vi "系统设置.vi"() -> ()   [LabVIEW 2016]
uses:
  PLC/control/switch.ctl
  <vilib>/Utility/miscctls.llb/LVPointTypeDef.ctl
  API/Alarm interface/interface.vi
  API/DGUS/SourceCode/DGUS/Interface/task.vi
  <vilib>/ptbypt/NI_PtbyPt.lvlib
  <vilib>/Utility/config.llb/NI_LVConfig.lvlib
  PLC/PLC.lvlib
  API/Alarm interface/Alarm interface.lvlib
  API/OpSignIn/opSignIn.lvlib
  API/DGUS/SourceCode/DGUS.lvlib
panel:
  in  "更新数据库密码":bool
  in  "性能测试模式":bool
  in  "运维打卡配置":bool
  in  "平行样测试":T1
  in  "采水模式":enum16{"单采水点", "交替采水"}(ring)
  in  "停止":T1
  in  "集成干预测试":T1
  out "最近一次启动时间":string
  in  "单次水样测试":T1
  in  "站点信息设置":bool
  in  "自动运行启动参数":T2
  in  "定时重启配置":bool
  in  "模块启用配置":bool
  in  "报警设置":bool
  in  "首页显示设置":bool
  in  "跨度核查":T1
  in  "零点核查":T1
  out "选项卡控件":enum32{"自由设定", "国标协议", "流量设定"}(tab)
  in  "24H周期设置":T3
  in  "采配水运行间隔":i16=4 min=0 max=24
  in  "多参数运行间隔":i16=4 min=0 max=24
  in  "湿化学运行间隔":i16=4 min=0 max=24
  in  "流量阈值":dbl=4.0 min=1.0 max=24.0
  in  "时间阈值":u16=4 min=1 max=24
  in  "周期设置":enum16{"自由设定", "国标协议", "流量设定"}(ring)
  in  "质控启动日期":string(combo)="关闭"
  in  "跨度核查时间":u16(ring)=6 items=["00H", "01H", "02H", "03H", "04H", "05H", "06H", "07H", "08H", "09H", "10H", "11H", "12H", "13H", "14H", "15H", "16H", "17H", "18H", "19H", "20H", "21H", "22H", "23H", "关闭"]
  in  "空白核查时间":u16(ring)=2 items=["00H", "01H", "02H", "03H", "04H", "05H", "06H", "07H", "08H", "09H", "10H", "11H", "12H", "13H", "14H", "15H", "16H", "17H", "18H", "19H", "20H", "21H", "22H", "23H", "关闭"]
  in  "副屏显示设置":bool
  in  "开机启动":bool caption="氨氮禁用"
  in  "运行模式":enum16{"维护模式", "常规模式", "应急模式", "质控模式"}(ring)
  # "注：周期设置分为自由设定和国标协议两种。\n1：选择自由设定情况下：运行间隔将不可选用并变灰色，周期设置可自由手动勾选\n2：选择国标协议情况下：周期时间将由运行间隔选择的时间决定，下方周期设置被禁用并无法手动勾选。\n3：选择流量设定情况下：瞬时流量连续超过流量阈值到达时间阈值设定值，仪器将自动开启测量。"
  # "质控频次："
  # "零点核查时间："
  # "跨度核查时间："
  # "启动周期设置"
  # "采水模式：\n单采水点：依据采水泵模式启动采水泵\n交替采水：采水泵根据周期设置交替启动"
  # "m3/S"
  # "秒"
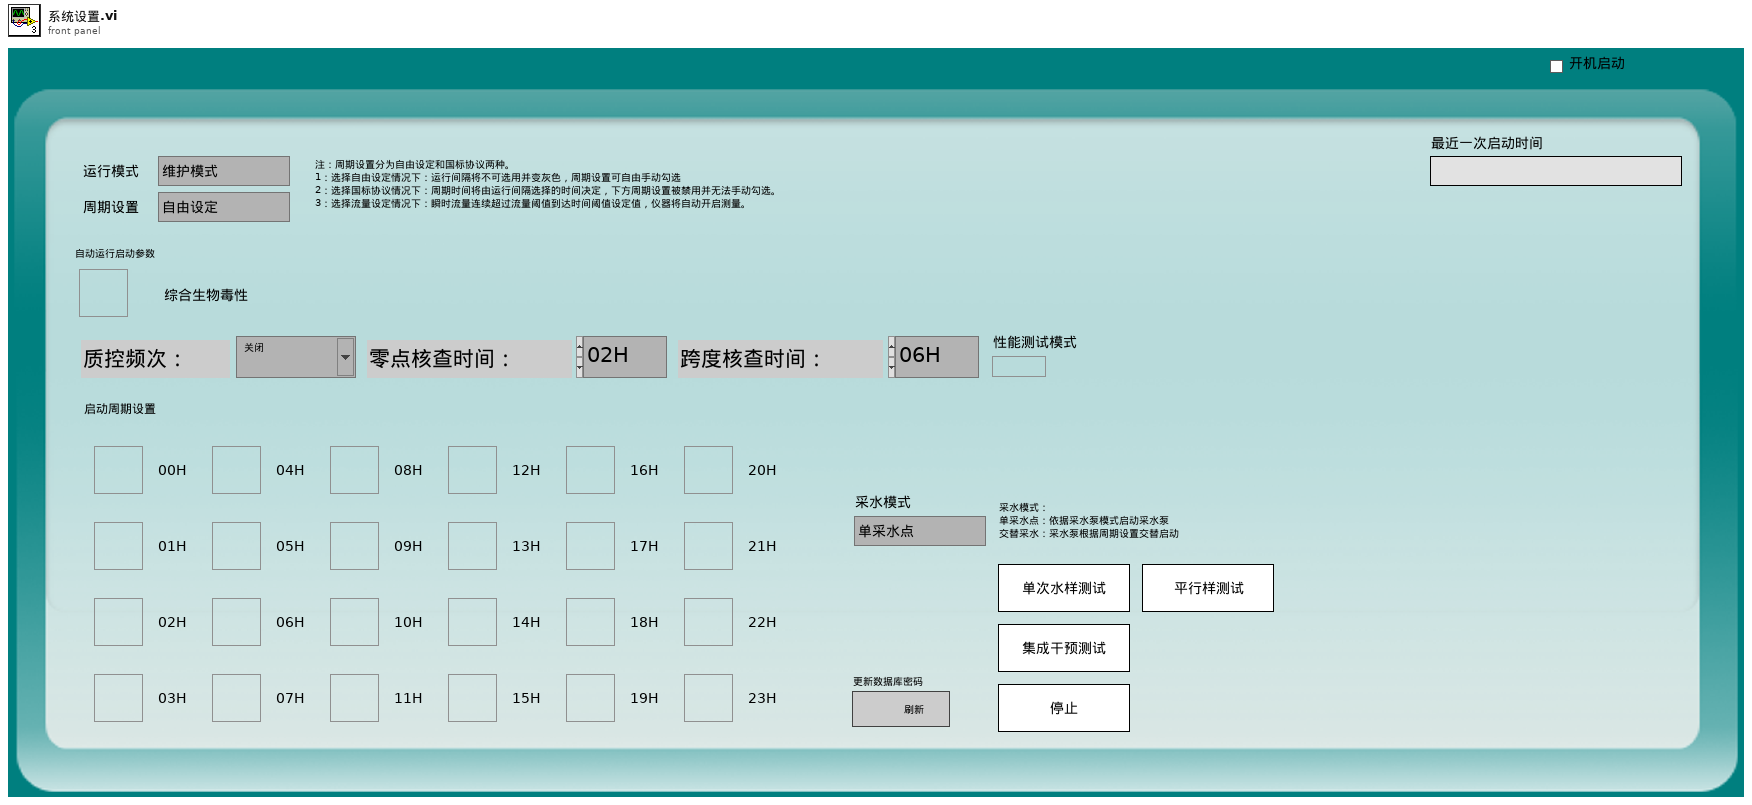
[diagram p1: front panel]
types:
  T1 = typedef "PLC.lvlib/switch.ctl" = bool
  T2 = typedef "启动参数.ctl" = cluster{"氨氮":bool, "总磷":bool, "总氮":bool, "多参数":bool, "CODmn":bool, "CODCr":bool, "氟化物":bool, "超标留样":bool, "重金属":bool, "挥发酚":bool, "综合生物毒性":bool}
  T3 = typedef "24周期设置.ctl" = cluster{"00H":bool, "01H":bool, "02H":bool, "03H":bool, "04H":bool, "05H":bool, "06H":bool, "07H":bool, "08H":bool, "09H":bool, "10H":bool, "11H":bool, "12H":bool, "13H":bool, "14H":bool, "15H":bool, "16H":bool, "17H":bool, "18H":bool, "19H":bool, "20H":bool, "21H":bool, "22H":bool, "23H":bool}
  T4 = cluster{"控制命令":enum16{"启动测量", "标样核查", "零点核查", "跨度核查", "空白测试", "平行样测试", "加标回收", "空白校准", "标样校准", "初始化（清洗）", "停止测试", "仪器重启", "校时", "模式设置", "测量间隔设置"}, "自动运行启动参数":T2}
  T5 = typedef "参数.ctl" = cluster{"测试模式":enum16{"水样测试", "平行样测试", "集成干预测试", "加标回收"}, "参数启用":T2}
  T6 = typedef "LVPointTypeDef.ctl" = cluster{"Horizontal":i16, "Vertical":i16}
  T7 = enum8{"Enabled", "Disabled", "Disabled and Grayed Out"}
  T8 = cluster{"频次":enum16{"关闭", "每天", "星期一", "星期二", "星期三", "星期四", "星期五", "星期六", "星期日"}, "时":u16, "分":u16}
  T9 = typedef "LVDateTimeRec.ctl" = cluster{"秒数的小数部分":dbl, "秒":i32, "分":i32, "时":i32, "日":i32, "月":i32, "年":i32, "天数（周）":i32, "天数（年）":i32, "DST":i32}
  T10 = enum16{"关闭", "每天", "星期一", "星期二", "星期三", "星期四", "星期五", "星期六", "星期日"}
  T11 = enum32{"Bad", "Idle", "Run top level", "Running"}
  T12 = enum32{"Invalid", "Standard", "Closed", "Hidden", "Minimized", "Maximized"}
  T13 = typedef "LVAllMonitorsDisplayTypeDef.ctl" = cluster{"Bounds":cluster{"Left":i16, "Top":i16, "Right":i16, "Bottom":i16}, "Depth":i16}[]
  T14 = cluster{"24H周期设置[0]":bool, "24H周期设置[1]":bool, "24H周期设置[2]":bool, "24H周期设置[3]":bool, "24H周期设置[4]":bool, "24H周期设置[5]":bool, "24H周期设置[6]":bool, "24H周期设置[7]":bool, "24H周期设置[8]":bool, "24H周期设置[9]":bool, "24H周期设置[10]":bool, "24H周期设置[11]":bool, "24H周期设置[12]":bool, "24H周期设置[13]":bool, "24H周期设置[14]":bool, "24H周期设置[15]":bool, "24H周期设置[16]":bool, "24H周期设置[17]":bool, "24H周期设置[18]":bool, "24H周期设置[19]":bool, "24H周期设置[20]":bool, "24H周期设置[21]":bool, "24H周期设置[22]":bool, "24H周期设置[23]":bool}
  T15 = typedef "操作日志字段定义.ctl" = cluster{"时间":timestamp, "参数":string, "日志信息":string, "流程参数":string}
  T16 = enum16{"启动测量", "标样核查", "零点核查", "跨度核查", "空白测试", "平行样测试", "加标回收", "空白校准", "标样校准", "初始化（清洗）", "停止测试", "仪器重启", "校时", "模式设置", "测量间隔设置"}
  T17 = cluster{"测试模式":enum16{"水样测试", "平行样测试", "集成干预测试", "加标回收"}, "启动参数输出":T2}
  T18 = typedef "NI_LVConfig.lvlib/Config Data RefNum.ctl" = refnum<k1>
  T19 = cluster{"元素":enum16{"启动测量", "标样核查", "零点核查", "跨度核查", "空白测试", "平行样测试", "加标回收", "空白校准", "标样校准", "初始化（清洗）", "停止测试", "仪器重启", "校时", "模式设置", "测量间隔设置"}, "启动参数输出":T2}
  T20 = cluster{"元素":enum16{"启动测量", "标样核查", "零点核查", "跨度核查", "空白测试", "平行样测试", "加标回收", "空白校准", "标样校准", "初始化（清洗）", "停止测试", "仪器重启", "校时", "模式设置", "测量间隔设置"}, "自动运行启动参数":T2}
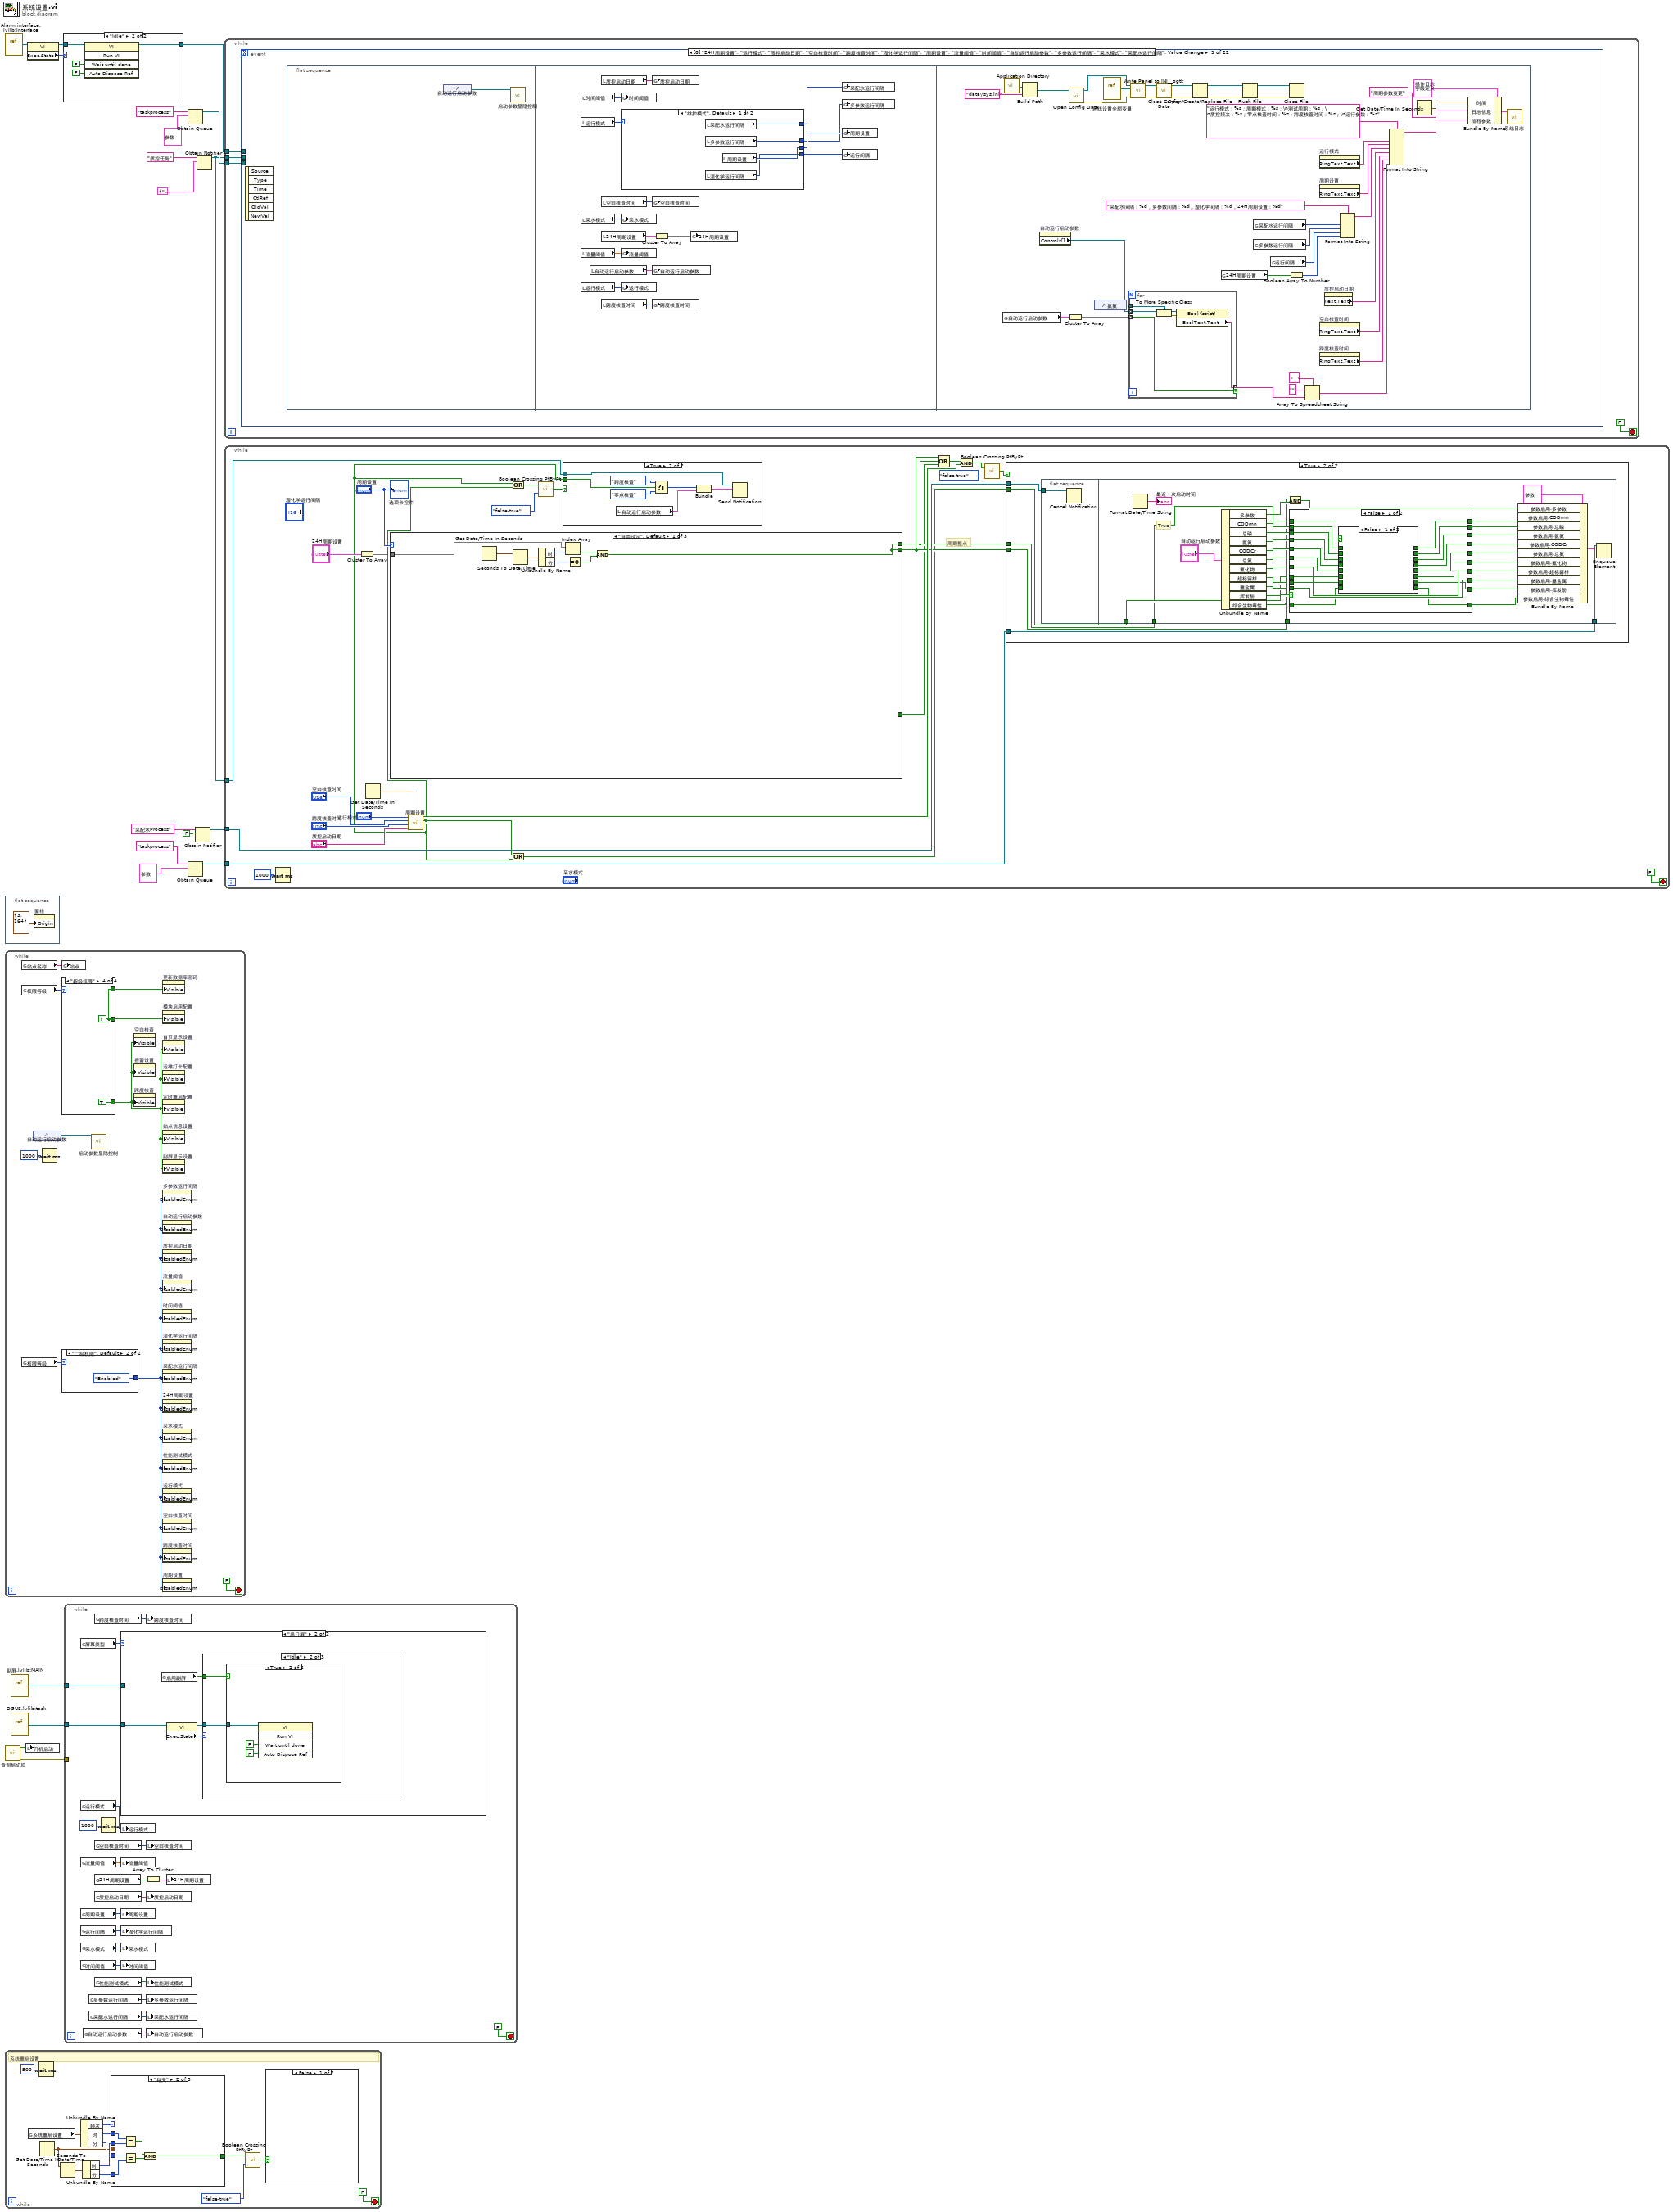
[diagram p0: block diagram]
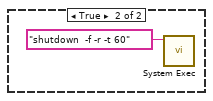
[diagram p2: hidden frame]
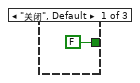
[diagram p3: hidden frame]
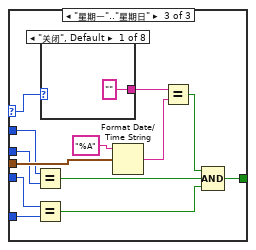
[diagram p4: hidden frame]
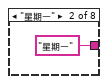
[diagram p5: hidden frame]
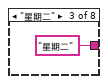
[diagram p6: hidden frame]
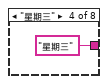
[diagram p7: hidden frame]
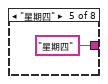
[diagram p8: hidden frame]
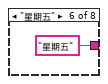
[diagram p9: hidden frame]
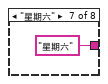
[diagram p10: hidden frame]
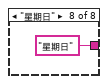
[diagram p11: hidden frame]
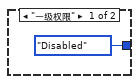
[diagram p13: hidden frame]
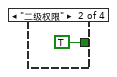
[diagram p15: hidden frame]
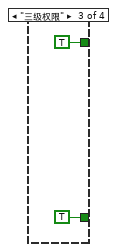
[diagram p16: hidden frame]
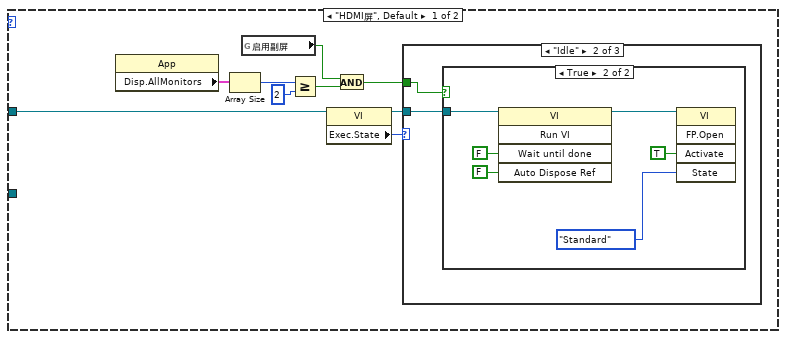
[diagram p17: hidden frame]
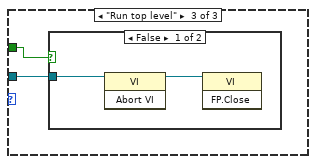
[diagram p20: hidden frame]
diagram:
  n1 = vi-ref "Alarm interface.lvlib:interface.vi"() -> (w15:refnum<vi>)
  n2 = flat-sequence {
    frame #0 {
      n3 = property on="窗格" class="Pane"("Origin"=T6 {"Horizontal"=3, "Vertical"=164} ("原点")) -> ()  [unwired: 2 in, 2 out]
    }
  }
  n4 = while {
    stop <- FALSE stop-if-true
    n5 = global read "非断电保持全局变量.vi" "站点名称"() -> (w28:string)
    n6 = global read "非断电保持全局变量.vi" "权限等级"() -> (w29:enum16{"一级权限", "二级权限", "三级权限", "超级权限"})
    n7 = global read "非断电保持全局变量.vi" "权限等级"() -> (w24:enum16{"一级权限", "二级权限", "三级权限", "超级权限"})
    n8 = control-ref of="自动运行启动参数"() -> (w25:refnum<vi>)
    n9 = Wait (ms)(milliseconds to wait=u32 1000 ("等待时间（毫秒）")) -> ()  [unwired: 1 out]
    n10 = global write "短信服务全局变量.vi" "站点"(w28) -> ()
    n11 = case shown="\"超级权限\"" w29 {
      tunnel: [_ TRUE TRUE TRUE] -> w26
      tunnel: [_ _ TRUE w37] -> w27
      tunnel: [_ _ _ w37] -> w22
      frame "一级权限", Default {
      }
      frame "二级权限" {
      }
      frame "三级权限" {
      }
      frame "超级权限" {
        w37 = TRUE
      }
    }
    n12 = case shown="\"二级权限\", Default" w24 {
      tunnel: [T7."Disabled" ("禁用") T7."Enabled" ("禁用")] -> w23
      frame "一级权限" {
      }
      frame "二级权限", Default {
      }
    }
    n13 = call "启动参数显隐控制.vi"("启动参数"=w25) -> ()  [unwired: 9 in, 1 out]
    n14 = property on="空白核查" class="Bool"("Visible"=w26) -> ()  [unwired: 2 in, 2 out]
    n15 = property on="报警设置" class="Bool"("Visible"=w26) -> ()  [unwired: 2 in, 2 out]
    n16 = property on="跨度核查" class="Bool"("Visible"=w26) -> ()  [unwired: 2 in, 2 out]
    n17 = property on="更新数据库密码" class="Bool"("Visible"=w22) -> ()  [unwired: 2 in, 2 out]
    n18 = property on="模块启用配置" class="Bool"("Visible"=w27) -> ()  [unwired: 2 in, 2 out]
    n19 = property on="首页显示设置" class="Bool"("Visible"=w26) -> ()  [unwired: 2 in, 2 out]
    n20 = property on="运维打卡配置" class="Bool"("Visible"=w26) -> ()  [unwired: 2 in, 2 out]
    n21 = property on="定时重启配置" class="Bool"("Visible"=w26) -> ()  [unwired: 2 in, 2 out]
    n22 = property on="站点信息设置" class="Bool"("Visible"=w26) -> ()  [unwired: 2 in, 2 out]
    n23 = property on="副屏显示设置" class="Bool"("Visible"=w26) -> ()  [unwired: 2 in, 2 out]
    n24 = property on="多参数运行间隔" class="DigNum (strict)"("DisabledEnum"=w23) -> ()  [unwired: 2 in, 2 out]
    n25 = property on="自动运行启动参数" class="Clust (strict)"("DisabledEnum"=w23) -> ()  [unwired: 2 in, 2 out]
    n26 = property on="质控启动日期" class="CmbBox"("DisabledEnum"=w23) -> ()  [unwired: 2 in, 2 out]
    n27 = property on="流量阈值" class="DigNum (strict)"("DisabledEnum"=w23) -> ()  [unwired: 2 in, 2 out]
    n28 = property on="时间阈值" class="DigNum (strict)"("DisabledEnum"=w23) -> ()  [unwired: 2 in, 2 out]
    n29 = property on="湿化学运行间隔" class="DigNum (strict)"("DisabledEnum"=w23) -> ()  [unwired: 2 in, 2 out]
    n30 = property on="采配水运行间隔" class="DigNum (strict)"("DisabledEnum"=w23) -> ()  [unwired: 2 in, 2 out]
    n31 = property on="24H周期设置" class="Clust (strict)"("DisabledEnum"=w23) -> ()  [unwired: 2 in, 2 out]
    n32 = property on="采水模式" class="Enum (strict)"("DisabledEnum"=w23) -> ()  [unwired: 2 in, 2 out]
    n33 = property on="性能测试模式" class="Bool (strict)"("DisabledEnum"=w23) -> ()  [unwired: 2 in, 2 out]
    n34 = property on="运行模式" class="Enum (strict)"("DisabledEnum"=w23) -> ()  [unwired: 2 in, 2 out]
    n35 = property on="空白核查时间" class="Ring (strict)"("DisabledEnum"=w23) -> ()  [unwired: 2 in, 2 out]
    n36 = property on="跨度核查时间" class="Ring (strict)"("DisabledEnum"=w23) -> ()  [unwired: 2 in, 2 out]
    n37 = property on="周期设置" class="Enum (strict)"("DisabledEnum"=w23) -> ()  [unwired: 2 in, 2 out]
  }
  n38 = call "查询启动项.vi"() -> ("error out"=w11:errorcluster, "包含启动项"=w17:bool)  [unwired: 10 in]
  n39 = while {
    stop <- FALSE stop-if-true
    # "系统重启设置"
    n40 = global read "系统设置全局变量.vi" "系统重启设置"() -> (w51:T8)
    n41 = Wait (ms)(milliseconds to wait=u32 500 ("等待时间（毫秒）")) -> ()  [unwired: 1 out]
    n42 = Get Date/Time In Seconds() -> (seconds since 1Jan1904=w42:timestamp)
    n43 = Seconds To Date/Time(time stamp (now)=w42) -> (date time rec=w49:T9)  [unwired: 1 in]
    n44 = Unbundle By Name(w51) -> ("频次"=w50:T10, "时"=w46:u16, "分"=w45:u16)
    n45 = Unbundle By Name(w49) -> ("时"=w48:i32, "分"=w47:i32)
    n46 = case shown="\"每天\"" w50 {
      selector: w50 -> [_ _ w71]
      tunnel: [FALSE w54 w61] -> w41
      tunnel: w48 -> [_ w60 w65]
      tunnel: w47 -> [_ w57 w63]
      tunnel: w46 -> [_ w59 w66]
      tunnel: w45 -> [_ w58 w64]
      tunnel: w42 -> [_ _ w72]
      frame "关闭", Default {
      }
      frame "每天" {
        n47 = Equal?(x=w59, y=w60) -> (x = y?=w55:bool)
        n48 = Equal?(x=w58, y=w57) -> (x = y?=w56:bool)
        n49 = And(x=w55, y=w56) -> (x .and. y?=w54:bool)
      }
      frame "星期一".."星期日" {
        n50 = Equal?(x=w66, y=w65) -> (x = y?=w67:bool)
        n51 = Equal?(x=w64, y=w63) -> (x = y?=w68:bool)
        n52 = case shown="\"关闭\", Default" w71 {
          tunnel: ["" ("时间格式字符串(%c)") "星期一" ("时间格式字符串(%c)") "星期二" ("时间格式字符串(%c)") "星期三" ("时间格式字符串(%c)") "星期四" ("时间格式字符串(%c)") "星期五" ("时间格式字符串(%c)") "星期六" ("时间格式字符串(%c)") "星期日" ("时间格式字符串(%c)")] -> w69
          frame "关闭", Default {
          }
          frame "星期一" {
          }
          frame "星期二" {
          }
          frame "星期三" {
          }
          frame "星期四" {
          }
          frame "星期五" {
          }
          frame "星期六" {
          }
          frame "星期日" {
          }
        }
        n53 = Format Date/Time String(time format string (%c)="%A" ("时间格式字符串(%c)"), seconds (now)=w72) -> (date/time string=w70:string)  [unwired: 1 in]
        n54 = Equal?(x=w69, y=w70) -> (x = y?=w62:bool)
        n55 = Compound Arithmetic op=AND ("复合运算")(w62, w67, w68) -> (w61:bool)
      }
    }
    n56 = call <vilib>:"Boolean Crossing PtByPt.vi"("direction"=enum16{"either", "false-true", "true-false"}."false-true", "input"=w41) -> ("crossing"=w39:bool)  [unwired: 1 in]
    n57 = case shown="False" w39 {
      frame False {
      }
      frame True {
        n58 = call <vilib>:"System Exec.vi"("command line"="shutdown  -f -r -t 60") -> ()  [unwired: 7 in, 4 out]
      }
    }
  }
  n59 = vi-ref "副屏.lvlib:MAIN.vi"() -> (w16:refnum<vi>)
  n60 = vi-ref "DGUS.lvlib:task.vi"() -> (w1:refnum<vi>)
  n61 = local write "开机启动"(w17) -> ()
  n62 = property class="VI"(reference=w15) -> (reference out=w13:refnum<vi>, "Exec.State"=w14:T11)  [unwired: 1 in, 1 out]
  n63 = case shown="\"Idle\"" w14 {
    tunnel: w13 -> [w82 w86]
    tunnel: [w82 w85] -> w12
    frame "Bad", Default {
    }
    frame "Idle" {
      n64 = invoke class="VI" method="Run VI"(reference=w86, "Wait until done"=FALSE ("结束前等待"), "Auto Dispose Ref"=FALSE ("自动销毁引用")) -> (reference out=w85:refnum<vi>)  [unwired: 2 in, 4 out]
    }
  }
  n65 = while {
    tunnel: w16 -> [w102]
    tunnel: w11 -> [_]
    tunnel: w1 -> [w88]
    stop <- FALSE stop-if-true
    n66 = global read "副屏设置全局变量.vi" "屏幕类型"() -> (w89:enum16{"HDMI屏", "串口屏"})
    n67 = global read "系统设置全局变量.vi" "运行模式"() -> (w96:enum16{"维护模式", "常规模式", "应急模式", "质控模式"})
    n68 = global read "系统设置全局变量.vi" "流量阈值"() -> (w95:dbl)
    n69 = global read "系统设置全局变量.vi" "周期设置"() -> (w98:enum16{"自由设定", "国标协议", "流量设定"})
    n70 = global read "系统设置全局变量.vi" "运行间隔"() -> (w97:i16)
    n71 = global read "系统设置全局变量.vi" "采水模式"() -> (w92:enum16{"单采水点", "交替采水"})
    n72 = global read "系统设置全局变量.vi" "时间阈值"() -> (w94:u16)
    n73 = global read "系统设置全局变量.vi" "自动运行启动参数"() -> (w103:T2)
    n74 = global read "系统设置全局变量.vi" "多参数运行间隔"() -> (w93:i16)
    n75 = global read "系统设置全局变量.vi" "采配水运行间隔"() -> (w90:i16)
    n76 = global read "系统设置全局变量.vi" "跨度核查时间"() -> (w99:u16)
    n77 = global read "系统设置全局变量.vi" "空白核查时间"() -> (w100:u16)
    n78 = global read "系统设置全局变量.vi" "24H周期设置"() -> (w104:bool[])
    n79 = global read "系统设置全局变量.vi" "质控启动日期"() -> (w101:string)
    n80 = global read "系统设置全局变量.vi" "性能测试模式"() -> (w87:bool)
    n81 = Wait (ms)(milliseconds to wait=u32 1000 ("等待时间（毫秒）")) -> ()  [unwired: 1 out]
    n82 = case shown="\"串口屏\"" w89 {
      tunnel: w102 -> [w115 _]
      tunnel: w88 -> [_ w131]
      frame "HDMI屏", Default {
        n83 = property class="App"() -> ("Disp.AllMonitors"=w111:T13)  [unwired: 2 in, 2 out]
        n84 = Array Size(array=w111) -> (size(s)=w107:i32)
        n85 = global read "副屏设置全局变量.vi" "启用副屏"() -> (w113:bool)
        n86 = Greater Or Equal?(x=w107, y=2) -> (x >= y?=w108:bool)
        n87 = property class="VI"(reference=w115) -> (reference out=w112:refnum<vi>, "Exec.State"=w114:T11)  [unwired: 1 in, 1 out]
        n88 = And(x=w113, y=w108) -> (x .and. y?=w109:bool)
        n89 = case shown="\"Idle\"" w114 {
          tunnel: w109 -> [_ w116 w124]
          tunnel: w112 -> [_ w117 w125]
          frame "Bad", Default {
          }
          frame "Idle" {
            n90 = case shown="True" w116 {
              tunnel: w117 -> [_ w123]
              frame False {
              }
              frame True {
                n91 = invoke class="VI" method="Run VI"(reference=w123, "Wait until done"=FALSE ("结束前等待"), "Auto Dispose Ref"=FALSE ("自动销毁引用")) -> (reference out=w118:refnum<vi>)  [unwired: 2 in, 4 out]
                n92 = invoke class="VI" method="FP.Open"(reference=w118, "Activate"=TRUE ("激活？"), "State"=T12."Standard" ("状态")) -> ()  [unwired: 2 in, 5 out]
              }
            }
          }
          frame "Run top level" {
            n93 = case shown="False" w124 {
              tunnel: w125 -> [w126 _]
              frame False {
                n94 = invoke class="VI" method="Abort VI"(reference=w126) -> (reference out=w127:refnum<vi>)  [unwired: 2 in, 2 out]
                n95 = invoke class="VI" method="FP.Close"(reference=w127) -> ()  [unwired: 2 in, 3 out]
              }
              frame True {
              }
            }
          }
        }
      }
      frame "串口屏" {
        n96 = global read "副屏设置全局变量.vi" "启用副屏"() -> (w129:bool)
        n97 = property class="VI"(reference=w131) -> (reference out=w128:refnum<vi>, "Exec.State"=w130:T11)  [unwired: 1 in, 1 out]
        n98 = case shown="\"Idle\"" w130 {
          tunnel: w129 -> [_ w132 _]
          tunnel: w128 -> [_ w133 _]
          frame "Bad", Default {
          }
          frame "Idle" {
            n99 = case shown="True" w132 {
              tunnel: w133 -> [_ w136]
              frame False {
              }
              frame True {
                n100 = invoke class="VI" method="Run VI"(reference=w136, "Wait until done"=FALSE ("结束前等待"), "Auto Dispose Ref"=FALSE ("自动销毁引用")) -> ()  [unwired: 2 in, 5 out]
              }
            }
          }
          frame "Running" {
          }
        }
      }
    }
    n101 = local write "运行模式"(w96) -> ()
    n102 = local write "流量阈值"(w95) -> ()
    n103 = local write "周期设置"(w98) -> ()
    n104 = local write "湿化学运行间隔"(w97) -> ()
    n105 = local write "采水模式"(w92) -> ()
    n106 = local write "时间阈值"(w94) -> ()
    n107 = Array To Cluster(array=w104) -> (cluster=w91:T14)
    n108 = local write "跨度核查时间"(w99) -> ()
    n109 = local write "空白核查时间"(w100) -> ()
    n110 = local write "质控启动日期"(w101) -> ()
    n111 = local write "性能测试模式"(w87) -> ()
    n112 = local write "多参数运行间隔"(w93) -> ()
    n113 = local write "采配水运行间隔"(w90) -> ()
    n114 = local write "自动运行启动参数"(w103) -> ()
    n115 = local write "24H周期设置"(w91) -> ()
  }
  n116 = Obtain Queue(name (unnamed)="taskprocess" ("名称（未命名）"), element data type=T5 {"测试模式"=enum."水样测试", "参数启用"={"氨氮"=FALSE, "总磷"=FALSE, "总氮"=FALSE, "多参数"=FALSE, "CODmn"=FALSE, "CODCr"=FALSE, "氟化物"=FALSE, "超标留样"=FALSE, "重金属"=FALSE, "挥发酚"=FALSE, "综合生物毒性"=FALSE}} ("参数")) -> (queue out=w7:refnum<queue>)  [unwired: 3 in, 2 out]
  n117 = Obtain Queue(name (unnamed)="taskprocess" ("名称（未命名）"), element data type=T5 {"测试模式"=enum."水样测试", "参数启用"={"氨氮"=FALSE, "总磷"=FALSE, "总氮"=FALSE, "多参数"=FALSE, "CODmn"=FALSE, "CODCr"=FALSE, "氟化物"=FALSE, "超标留样"=FALSE, "重金属"=FALSE, "挥发酚"=FALSE, "综合生物毒性"=FALSE}} ("参数")) -> (queue out=w9:refnum<queue>)  [unwired: 3 in, 2 out]
  n118 = Obtain Notifier(name (unnamed)="采配水Process" ("名称（未命名）"), notification data type=FALSE) -> (notifier out=w18:refnum<notifier>)  [unwired: 2 in, 2 out]
  n119 = Obtain Notifier(name (unnamed)="质控任务" ("名称（未命名）"), notification data type=T4 {"控制命令"=enum."启动测量", "自动运行启动参数"={"氨氮"=FALSE, "总磷"=FALSE, "总氮"=FALSE, "多参数"=FALSE, "CODmn"=FALSE, "CODCr"=FALSE, "氟化物"=FALSE, "超标留样"=FALSE, "重金属"=FALSE, "挥发酚"=FALSE, "综合生物毒性"=FALSE}}) -> (notifier out=w2:refnum<notifier>)  [unwired: 2 in, 2 out]
  n120 = while {
    tunnel: w12 -> [w139]
    tunnel: w7 -> [w138]
    tunnel: w2 -> [w137]
    stop <- FALSE stop-if-true
    n121 = event shown="[8] \"24H周期设置\", \"运行模式\", \"质控启动日期\", \"空白核查时间\", \"跨度核查时间\", \"湿化学运行间隔\", \"周期设置\", \"流量阈值\", \"时间阈值\", \"自动运行启动参数\", \"多参数运行间隔\", \"采水模式\", \"采配水运行间隔\": Value Change" {
      selector: _ -> [_ _ _ _ _ _ _ _ _ _ _ _ _ _ _ _ _ _ _ _ _ _]
      dyn-events: _ -> [_ _ _ _ _ _ _ _ _ _ _ _ _ _ _ _ _ _ _ _ _ _]
      timeout: _ -> [_ _ _ _ _ _ _ _ _ _ _ _ _ _ _ _ _ _ _ _ _ _]
      tunnel: w139 -> [_ _ _ _ _ _ _ _ _ _ _ _ _ _ _ _ _ w300 _ _ _ _]
      tunnel: w138 -> [_ _ w143 _ _ _ _ _ _ _ _ _ _ _ _ _ _ _ w303 _ _ w324]
      tunnel: w137 -> [_ _ _ _ _ _ _ _ _ _ _ _ _ _ _ _ _ _ _ w308 w315 _]
      event Timeout {
        n122 = event-data() -> ()  [unwired: 1 in, 3 out]
      }
      event Value Change {
        n123 = event-data() -> ()  [unwired: 1 in, 6 out]
        n124 = call "停止流程.vi"() -> ()  [unwired: 12 in]
      }
      event Value Change {
        n125 = event-data() -> ()  [unwired: 1 in, 6 out]
        n126 = call "启动参数选择.vi"() -> ("check？"=w141:bool, "启动参数输出"=w142:T2)  [unwired: 10 in]
        n127 = case shown="True" w141 {
          tunnel: w143 -> [_ w147]
          tunnel: w142 -> [_ w144]
          frame False {
          }
          frame True {
            n128 = Bundle("测试模式"=enum16{"水样测试", "平行样测试", "集成干预测试", "加标回收"}."水样测试", "启动参数输出"=w144) -> (w145:T17)  [unwired: 1 in]
            n129 = Enqueue Element(queue=w147, element=w145) -> ()  [unwired: 2 in, 3 out]
          }
        }
      }
      event "站点信息设置": Value Change {
        n130 = event-data() -> ()  [unwired: 1 in, 6 out]
        n131 = call "站点信息设置.vi"() -> ()  [unwired: 12 in]
      }
      event "运维打卡配置": Value Change {
        n132 = event-data() -> ()  [unwired: 1 in, 6 out]
        n133 = call "配置对话框.vi"() -> ()  [unwired: 12 in]
      }
      event "定时重启配置": Value Change {
        n134 = event-data() -> ()  [unwired: 1 in, 6 out]
        n135 = call "重启设置.vi"() -> ()  [unwired: 12 in]
      }
      event "模块启用配置": Value Change {
        n136 = event-data() -> ()  [unwired: 1 in, 6 out]
        n137 = call "模块启用配置框.vi"() -> ()  [unwired: 12 in]
      }
      event "更新数据库密码": Value Change {
        n138 = event-data() -> ()  [unwired: 1 in, 6 out]
        n139 = call "读取秘钥.vi"() -> ("error out"=w152:errorcluster, "值"=w153:string[])  [unwired: 9 in, 1 out]
        n140 = call "Generate_random_password.vi"("error in (no error)"=w152) -> ("error out"=w154:errorcluster, "Generate random password"=w149:string)  [unwired: 9 in]
        n141 = Index Array(array=w153) -> (element=w151:string)  [unwired: 1 in]
        n142 = Bundle("Generate random password"=w149) -> (w155:cluster{"Generate random password":string})  [unwired: 1 in]
        n143 = call "添加秘钥.vi"("error in (no error)"=w154, "簇"=w155) -> ("error out"=w150:errorcluster, "添加成功标记"=w148:bool)  [unwired: 8 in]
        n144 = case shown="True" w148 {
          tunnel: w149 -> [_ w171]
          frame False {
            n145 = One Button Dialog(message="数据库秘钥更新失败!" ("消息")) -> ()  [unwired: 1 in, 1 out]
          }
          frame True {
            n146 = global write "外部调用接口全局变量.vi" "Password"(w171) -> ()
            n147 = global write "非断电保持全局变量.vi" "Password"(w171) -> ()
            n148 = One Button Dialog(message="数据库秘钥更新成功!" ("消息")) -> ()  [unwired: 1 in, 1 out]
          }
        }
        n149 = case shown="True" w148 {
          tunnel: w151 -> [_ w157]
          tunnel: w150 -> [_ w169]
          tunnel: w149 -> [_ w168]
          frame False {
          }
          frame True {
            n150 = call "database path.vi"("database"="database1") -> ("Path out"=w166:string)  [unwired: 9 in, 1 out]
            n151 = String To Path(string=w166) -> (path=w165:path)
            n152 = call "alter database password.vi"("错误输入（无错误）"=w169, "NewPWd"=w168, "OpenPwd"=w157, "路径"=w165) -> ("错误输出"=w161:errorcluster)  [unwired: 7 in]
            n153 = call "database path.vi"("database"="database3") -> ("Path out"=w163:string)  [unwired: 9 in, 1 out]
            n154 = call <vilib>:"Clear Errors.vi"("error in (no error)"=w161) -> ("error out"=w160:errorcluster)  [unwired: 5 in, 1 out]
            n155 = String To Path(string=w163) -> (path=w164:path)
            n156 = call "alter database password.vi"("错误输入（无错误）"=w160, "NewPWd"=w168, "OpenPwd"=w157, "路径"=w164) -> ()  [unwired: 7 in, 1 out]
            n157 = Concatenate Strings("Old_password:" ("字符串"), w157, "New_password:*********" ("字符串")) -> (w156:string)
            n158 = call "Password_Log写入.vi"("Log"=w156) -> ()  [unwired: 11 in]
          }
        }
      }
      event "运行模式", "质控启动日期", "空白核查时间", "跨度核查时间", "湿化学运行间隔", "周期设置", "流量阈值", "时间阈值", "多参数运行间隔", "采水模式", "采配水运行间隔": Value Change {
        n159 = event-data() -> ()  [unwired: 1 in, 6 out]
        n160 = flat-sequence {
          frame #0 {
            n161 = control-ref of="自动运行启动参数"() -> (w173:refnum<vi>)
            n162 = call "启动参数显隐控制.vi"("启动参数"=w173) -> ()  [unwired: 9 in, 1 out]
          }
          frame #1 {
            n163 = local read "时间阈值"() -> (w183:u16)
            n164 = local read "运行模式"() -> (w178:enum16{"维护模式", "常规模式", "应急模式", "质控模式"})
            n165 = local read "采水模式"() -> (w180:enum16{"单采水点", "交替采水"})
            n166 = local read "流量阈值"() -> (w182:dbl)
            n167 = local read "运行模式"() -> (w188:enum16{"维护模式", "常规模式", "应急模式", "质控模式"})
            n168 = local read "自动运行启动参数"() -> (w181:T2)
            n169 = local read "质控启动日期"() -> (w186:string)
            n170 = local read "空白核查时间"() -> (w185:u16)
            n171 = local read "24H周期设置"() -> (w187:T3)
            n172 = local read "跨度核查时间"() -> (w184:u16)
            n173 = global write "系统设置全局变量.vi" "时间阈值"(w183) -> ()
            n174 = case shown="\"维护模式\", Default" w178 {
              tunnel: [w192 enum16{"自由设定", "国标协议", "流量设定"}."国标协议" ("周期设置")] -> w177
              tunnel: [w191 i16 1 ("多参数运行间隔")] -> w176
              tunnel: [w190 i16 1 ("多参数运行间隔")] -> w175
              tunnel: [w189 i16 0 ("多参数运行间隔")] -> w174
              frame "维护模式", Default {
                n175 = local read "采配水运行间隔"() -> (w189:i16)
                n176 = local read "多参数运行间隔"() -> (w190:i16)
                n177 = local read "湿化学运行间隔"() -> (w191:i16)
                n178 = local read "周期设置"() -> (w192:enum16{"自由设定", "国标协议", "流量设定"})
              }
              frame "应急模式" {
              }
            }
            n179 = global write "系统设置全局变量.vi" "采水模式"(w180) -> ()
            n180 = global write "系统设置全局变量.vi" "流量阈值"(w182) -> ()
            n181 = global write "系统设置全局变量.vi" "运行模式"(w188) -> ()
            n182 = global write "系统设置全局变量.vi" "质控启动日期"(w186) -> ()
            n183 = global write "系统设置全局变量.vi" "空白核查时间"(w185) -> ()
            n184 = global write "系统设置全局变量.vi" "自动运行启动参数"(w181) -> ()
            n185 = global write "系统设置全局变量.vi" "跨度核查时间"(w184) -> ()
            n186 = Cluster To Array(cluster=w187) -> (array=w179:bool[])
            n187 = global write "系统设置全局变量.vi" "24H周期设置"(w179) -> ()
            n188 = global write "系统设置全局变量.vi" "采配水运行间隔"(w174) -> ()
            n189 = global write "系统设置全局变量.vi" "多参数运行间隔"(w175) -> ()
            n190 = global write "系统设置全局变量.vi" "周期设置"(w177) -> ()
            n191 = global write "系统设置全局变量.vi" "运行间隔"(w176) -> ()
          }
          frame #2 {
            n192 = global read "系统设置全局变量.vi" "自动运行启动参数"() -> (w204:T2)
            n193 = call <vilib>:"Application Directory.vi"() -> ("Application Directory"=w236:path)
            n194 = Build Path(base path=w236, name or relative path="data\\sys.ini" ("名称或相对路径")) -> (appended path=w234:path)
            n195 = property on="自动运行启动参数" class="Clust (strict)"() -> ("Controls[]"=w202:refnum<vi>[])  [unwired: 2 in, 2 out]
            n196 = Cluster To Array(cluster=w204) -> (array=w203:bool[])
            n197 = call <vilib>:"Open Config Data.vi"("configuration file path"=w234) -> ("error out"=w230:errorcluster, "refnum"=w233:T18)  [unwired: 8 in, 1 out]
            n198 = control-ref of="氨氮"() -> (w201:refnum<vi>)
            n199 = vi-ref "系统设置全局变量.vi"() -> (w232:refnum<vi>)
            n200 = for {
              tunnel: w203 -> [w237] mode=indexing
              tunnel: w202 -> [w242] mode=indexing
              tunnel: w201 -> [w241]
              tunnel: [w238] -> w200 mode=indexing if=w237
              n201 = To More Specific Class(target class=w241, reference=w242) -> (specific class reference=w240:refnum<vi>, error out=w239:errorcluster)  [unwired: 1 in]
              n202 = property class="Bool (strict)"(reference=w240, error in=w239) -> ("BoolText.Text"=w238:string)  [unwired: 2 out]
            }
            n203 = call <userlib>:"Write Panel to INI__ogtk.vi"("error in (no error)"=w230, "VI ref"=w232, "refnum"=w233) -> ("error out"=w229:errorcluster, "refnum out"=w231:T18)  [unwired: 7 in]
            n204 = call <vilib>:"Close Config Data.vi"("error in (no error)"=w229, "refnum"=w231) -> ("error out"=w224:errorcluster, "file path"=w223:path)  [unwired: 8 in]
            n205 = Open/Create/Replace File(file path (use dialog)=w223, error in=w224) -> (refnum out=w227:refnum<file>, error out=w228:errorcluster)  [unwired: 4 in, 1 out]
            n206 = global read "系统设置全局变量.vi" "24H周期设置"() -> (w209:bool[])
            n207 = Flush File(refnum=w227, error in=w228) -> (refnum out=w226:refnum<file>, error out=w225:errorcluster)
            n208 = global read "系统设置全局变量.vi" "采配水运行间隔"() -> (w212:i16)
            n209 = global read "系统设置全局变量.vi" "多参数运行间隔"() -> (w211:i16)
            n210 = global read "系统设置全局变量.vi" "运行间隔"() -> (w210:i16)
            n211 = Close File(refnum=w226, error in=w225) -> ()  [unwired: 2 out]
            n212 = Boolean Array To Number(Boolean array=w209) -> (number=w208:u32)
            n213 = Array To Spreadsheet String(delimiter (Tab)="，" ("分隔符(Tab)"), array=w200, 3:"" ("格式字符串")) -> (spreadsheet string=w197:string)
            n214 = property on="运行模式" class="Enum (strict)"() -> ("RingText.Text"=w217:string)  [unwired: 2 in, 2 out]
            n215 = property on="周期设置" class="Enum (strict)"() -> ("RingText.Text"=w216:string)  [unwired: 2 in, 2 out]
            n216 = property on="空白核查时间" class="Ring (strict)"() -> ("RingText.Text"=w206:string)  [unwired: 2 in, 2 out]
            n217 = property on="跨度核查时间" class="Ring (strict)"() -> ("RingText.Text"=w205:string)  [unwired: 2 in, 2 out]
            n218 = property on="质控启动日期" class="CmbBox"() -> ("Text.Text"=w207:string)  [unwired: 2 in, 2 out]
            n219 = Format Into String(format string="采配水间隔：%d，多参数间隔：%d，湿化学间隔：%d，24H周期设置：%d" ("格式字符串"), w212, w211, w210, w208) -> (resulting string=w214:string)  [unwired: 2 in, 1 out]
            n220 = Format Into String(format string="运行模式：%s；周期模式：%s；\n测试周期：%s；\n质控频次：%s；零点核查时间：%s；跨度核查时间：%s；\n运行参数：%s" ("格式字符串"), w217, w216, w214, w207, w206, w205, w197) -> (resulting string=w218:string)  [unwired: 2 in, 1 out]
            n221 = Get Date/Time In Seconds() -> (seconds since 1Jan1904=w220:timestamp)
            n222 = Bundle By Name(cluster=T15 {"时间"=timestamp(0 s since 1904-01-01), "参数"="系统", "日志信息"="", "流程参数"=""} ("data in"), "时间"=w220, "日志信息"="周期参数变更", "流程参数"=w218) -> (w221:T15)
            n223 = call "系统日志.vi"("data in"=w221) -> ()  [unwired: 11 in]
          }
        }
      }
      event "性能测试模式": Value Change {
        n224 = event-data() -> ("OldVal"=w244:bool)  [unwired: 1 in]
        n225 = case shown="False" w244 {
          tunnel: [w260 _] -> w243
          frame False {
            n226 = Two Button Dialog(message="请确认是否切换为性能测试模式，在此模式下，所有数据的测试标识都将变更为PF!" ("消息")) -> (T button?=w261:bool)  [unwired: 2 in]
            n227 = case shown="True" w261 {
              tunnel: [_ TRUE] -> w260
              frame False {
              }
              frame True {
              }
            }
          }
          frame True {
          }
        }
        n228 = flat-sequence {
          tunnel: w243 -> [w245]
          frame #0 {
            n229 = global write "系统设置全局变量.vi" "性能测试模式"(w245) -> ()
          }
          frame #1 {
            n230 = call <vilib>:"Application Directory.vi"() -> ("Application Directory"=w246:path)
            n231 = Build Path(base path=w246, name or relative path="data\\sys.ini" ("名称或相对路径")) -> (appended path=w248:path)
            n232 = call <vilib>:"Open Config Data.vi"("configuration file path"=w248) -> ("error out"=w252:errorcluster, "refnum"=w249:T18)  [unwired: 8 in, 1 out]
            n233 = vi-ref "系统设置全局变量.vi"() -> (w250:refnum<vi>)
            n234 = call <userlib>:"Write Panel to INI__ogtk.vi"("error in (no error)"=w252, "VI ref"=w250, "refnum"=w249) -> ("error out"=w253:errorcluster, "refnum out"=w251:T18)  [unwired: 7 in]
            n235 = call <vilib>:"Close Config Data.vi"("error in (no error)"=w253, "refnum"=w251) -> ("error out"=w258:errorcluster, "file path"=w259:path)  [unwired: 8 in]
            n236 = Open/Create/Replace File(file path (use dialog)=w259, error in=w258) -> (refnum out=w255:refnum<file>, error out=w254:errorcluster)  [unwired: 4 in, 1 out]
            n237 = Flush File(refnum=w255, error in=w254) -> (refnum out=w256:refnum<file>, error out=w257:errorcluster)
            n238 = Close File(refnum=w256, error in=w257) -> ()  [unwired: 2 out]
          }
        }
      }
      event "湿化学运行间隔", "多参数运行间隔", "采配水运行间隔": Mouse Down {
        n239 = event-data() -> ("CtlRef"=w266:refnum<vi>)  [unwired: 1 in, 7 out]
        n240 = property class="DigNum (strict)"(reference=w266) -> (reference out=w265:refnum<vi>, "DisabledEnum"=w264:T7)  [unwired: 1 in, 1 out]
        n241 = case shown="\"Enabled\", Default" w264 {
          tunnel: w265 -> [w267 _]
          frame "Enabled", Default {
            n242 = property class="DigNum (strict)"(reference=w267) -> (reference out=w270:refnum<vi>, "Value"=w269:i16)  [unwired: 1 in, 1 out]
            n243 = call "数字键盘.vi"("OldNumber"=w269) -> ("NewNumber"=w268:sgl)
            n244 = property class="DigNum (strict)"(reference=w270, "Val(Sgnl)"=w268) -> ()  [unwired: 1 in, 2 out]
          }
          frame "Disabled" {
            n245 = One Button Dialog(message="权限不足，请提升操作权限！" ("消息")) -> ()  [unwired: 1 in, 1 out]
          }
        }
      }
      event "流量阈值": Mouse Down {
        n246 = event-data() -> ("CtlRef"=w272:refnum<vi>)  [unwired: 1 in, 7 out]
        n247 = property class="DigNum (strict)"(reference=w272) -> (reference out=w274:refnum<vi>, "DisabledEnum"=w273:T7)  [unwired: 1 in, 1 out]
        n248 = case shown="\"Enabled\", Default" w273 {
          tunnel: w274 -> [w275 _]
          frame "Enabled", Default {
            n249 = property class="DigNum (strict)"(reference=w275) -> (reference out=w278:refnum<vi>, "Value"=w277:dbl)  [unwired: 1 in, 1 out]
            n250 = call "数字键盘.vi"("OldNumber"=w277) -> ("NewNumber"=w276:sgl)
            n251 = property class="DigNum (strict)"(reference=w278, "Val(Sgnl)"=w276) -> ()  [unwired: 1 in, 2 out]
          }
          frame "Disabled" {
            n252 = One Button Dialog(message="权限不足，请提升操作权限！" ("消息")) -> ()  [unwired: 1 in, 1 out]
          }
        }
      }
      event "时间阈值": Mouse Down {
        n253 = event-data() -> ("CtlRef"=w280:refnum<vi>)  [unwired: 1 in, 7 out]
        n254 = property class="DigNum (strict)"(reference=w280) -> (reference out=w282:refnum<vi>, "DisabledEnum"=w281:T7)  [unwired: 1 in, 1 out]
        n255 = case shown="\"Disabled\"" w281 {
          tunnel: w282 -> [w283 _]
          frame "Enabled", Default {
            n256 = property class="DigNum (strict)"(reference=w283) -> (reference out=w286:refnum<vi>, "Value"=w285:u16)  [unwired: 1 in, 1 out]
            n257 = call "数字键盘.vi"("OldNumber"=w285) -> ("NewNumber"=w284:sgl)
            n258 = property class="DigNum (strict)"(reference=w286, "Val(Sgnl)"=w284) -> ()  [unwired: 1 in, 2 out]
          }
          frame "Disabled" {
            n259 = One Button Dialog(message="权限不足，请提升操作权限！" ("消息")) -> ()  [unwired: 1 in, 1 out]
          }
        }
      }
      event "运行模式", "空白核查时间", "跨度核查时间", "质控启动日期", "周期设置", "采水模式", "性能测试模式": Mouse Down {
        n260 = event-data() -> ("CtlRef"=w288:refnum<vi>)  [unwired: 1 in, 7 out]
        n261 = property class="Ctl"(reference=w288) -> ("DisabledEnum"=w289:T7)  [unwired: 1 in, 2 out]
        n262 = case shown="\"Disabled\"" w289 {
          frame "Enabled", Default {
          }
          frame "Disabled" {
            n263 = One Button Dialog(message="权限不足，请提升操作权限！" ("消息")) -> ()  [unwired: 1 in, 1 out]
          }
        }
      }
      event "开机启动": Value Change {
        n264 = event-data() -> ("NewVal"=w291:bool)  [unwired: 1 in, 5 out]
        n265 = case shown="False" w291 {
          frame False {
            n266 = call "删除启动项.vi"() -> ("删除标记"=w292:bool)  [unwired: 10 in, 1 out]
            n267 = case shown="False" w292 {
              frame False {
                n268 = local write "开机启动"(TRUE ("开机启动")) -> ()
                n269 = One Button Dialog(message="启动项删除失败" ("消息")) -> ()  [unwired: 1 in, 1 out]
              }
              frame True {
              }
            }
          }
          frame True {
            n270 = call "添加启动项.vi"() -> ("添加成功标记"=w295:bool)  [unwired: 10 in, 1 out]
            n271 = case shown="False" w295 {
              frame False {
                n272 = local write "开机启动"(FALSE ("开机启动")) -> ()
                n273 = One Button Dialog(message="启动项添加失败" ("消息")) -> ()  [unwired: 1 in, 1 out]
              }
              frame True {
              }
            }
          }
        }
      }
      event "副屏显示设置": Value Change {
        n274 = event-data() -> ()  [unwired: 1 in, 6 out]
        n275 = call "副屏设置.vi"() -> ()  [unwired: 12 in]
      }
      event "首页显示设置": Value Change {
        n276 = event-data() -> ()  [unwired: 1 in, 6 out]
        n277 = call "首页显示设置.vi"() -> ()  [unwired: 12 in]
      }
      event "报警设置": Value Change {
        n278 = event-data() -> ()  [unwired: 1 in, 6 out]
        n279 = invoke class="VI" method="FP.Open"(reference=w300, "Activate"=TRUE ("激活？"), "State"=T12."Standard" ("状态")) -> ()  [unwired: 2 in, 5 out]
      }
      event Value Change {
        n280 = event-data() -> ()  [unwired: 1 in, 6 out]
        n281 = call "启动参数选择.vi"() -> ("check？"=w301:bool, "启动参数输出"=w302:T2)  [unwired: 10 in]
        n282 = case shown="True" w301 {
          tunnel: w303 -> [_ w305]
          tunnel: w302 -> [_ w304]
          frame False {
          }
          frame True {
            n283 = Bundle("测试模式"=enum16{"水样测试", "平行样测试", "集成干预测试", "加标回收"}."集成干预测试", "启动参数输出"=w304) -> (w306:T17)  [unwired: 1 in]
            n284 = Enqueue Element(queue=w305, element=w306) -> ()  [unwired: 2 in, 3 out]
          }
        }
      }
      event Value Change {
        n285 = event-data() -> ()  [unwired: 1 in, 6 out]
        n286 = call "启动参数选择.vi"() -> ("check？"=w309:bool, "启动参数输出"=w310:T2)  [unwired: 10 in]
        n287 = case shown="True" w309 {
          tunnel: w310 -> [_ w314]
          tunnel: w308 -> [_ w312]
          frame False {
          }
          frame True {
            n288 = Bundle("元素"=T16."零点核查", "启动参数输出"=w314) -> (w311:T19)  [unwired: 1 in]
            n289 = Send Notification(notification=w311, notifier=w312) -> ()  [unwired: 1 in, 2 out]
          }
        }
      }
      event Value Change {
        n290 = event-data() -> ()  [unwired: 1 in, 6 out]
        n291 = call "启动参数选择.vi"() -> ("check？"=w316:bool, "启动参数输出"=w317:T2)  [unwired: 10 in]
        n292 = case shown="True" w316 {
          tunnel: w317 -> [_ w321]
          tunnel: w315 -> [_ w319]
          frame False {
          }
          frame True {
            n293 = Bundle("元素"=T16."跨度核查", "启动参数输出"=w321) -> (w318:T19)  [unwired: 1 in]
            n294 = Send Notification(notification=w318, notifier=w319) -> ()  [unwired: 1 in, 2 out]
          }
        }
      }
      event Value Change {
        n295 = event-data() -> ()  [unwired: 1 in, 6 out]
        n296 = call "启动参数选择.vi"() -> ("check？"=w322:bool, "启动参数输出"=w323:T2)  [unwired: 10 in]
        n297 = case shown="True" w322 {
          tunnel: w324 -> [_ w326]
          tunnel: w323 -> [_ w325]
          frame False {
          }
          frame True {
            n298 = Bundle("测试模式"=enum16{"水样测试", "平行样测试", "集成干预测试", "加标回收"}."平行样测试", "启动参数输出"=w325) -> (w327:T17)  [unwired: 1 in]
            n299 = Enqueue Element(queue=w326, element=w327) -> ()  [unwired: 2 in, 3 out]
          }
        }
      }
    }
  }
  n300 = while {
    tunnel: w18 -> [w353]
    tunnel: w9 -> [w347]
    tunnel: w2 -> [w338]
    stop <- FALSE stop-if-true
    # "周期整点"
    n301 = Wait (ms)(milliseconds to wait=u32 1000 ("等待时间（毫秒）")) -> ()  [unwired: 1 out]
    n302 = Cluster To Array(cluster="24H周期设置") -> (array=w331:bool[])
    n303 = Get Date/Time In Seconds() -> (seconds since 1Jan1904=w341:timestamp)
    n304 = case shown="\"自由设定\", Default" "周期设置" {
      tunnel: [w356 w387 w411] -> w335
      tunnel: w331 -> [w357 w388 _]
      tunnel: [w356 w376 w411] -> w336
      tunnel: [_ w364 _] -> w329
      frame "自由设定", Default {
        n305 = Get Date/Time In Seconds() -> (seconds since 1Jan1904=w358:timestamp)
        n306 = Seconds To Date/Time(time stamp (now)=w358) -> (date time rec=w359:T9)  [unwired: 1 in]
        n307 = Unbundle By Name(w359) -> ("时"=w362:i32, "分"=w360:i32)
        n308 = Index Array(array=w357, index=w362) -> (element=w363:bool)
        n309 = Equal To 0?(x=w360) -> (x = 0?=w361:bool)
        n310 = And(x=w363, y=w361) -> (x .and. y?=w356:bool)
      }
      frame "国标协议" {
        n311 = Get Date/Time In Seconds() -> (seconds since 1Jan1904=w389:timestamp)
        n312 = local read "湿化学运行间隔"() -> (w398:i16)
        n313 = Seconds To Date/Time(time stamp (now)=w389) -> (date time rec=w390:T9)  [unwired: 1 in]
        n314 = Unbundle By Name(w390) -> ("时"=w393:i32, "分"=w391:i32)
        n315 = call "运行间隔计算.vi"("运行周期"=w398) -> ("数组"=w397:i32[])  [unwired: 10 in]
        n316 = Index Array(array=w388, index=w393) -> (element=w394:bool)
        n317 = Equal To 0?(x=w391) -> (x = 0?=w392:bool)
        n318 = And(x=w394, y=w392) -> (x .and. y?=w387:bool)
        n319 = call "运行间隔计算.vi"("运行周期"="多参数运行间隔") -> ("数组"=w379:i32[])  [unwired: 10 in]
        n320 = call "运行间隔计算.vi"("运行周期"="采配水运行间隔") -> ("数组"=w373:i32[])  [unwired: 10 in]
        n321 = for {
          tunnel: w397 -> [w409] mode=indexing
          shift-right: [w407] -> w395
          shift-left: bool[] [FALSE, FALSE, FALSE, FALSE, FALSE, FALSE, FALSE, FALSE, FALSE, FALSE, FALSE, FALSE, FALSE, FALSE, FALSE, FALSE, FALSE, FALSE, FALSE, FALSE, FALSE, FALSE, FALSE, FALSE] ("24H周期设置") -> [w410]
          n322 = Replace Array Subset(array=w410, new element=TRUE ("新元素/子数组"), index=w409) -> (w407:bool[])
        }
        n323 = for {
          tunnel: w379 -> [w405] mode=indexing
          shift-right: [w403] -> w378
          shift-left: bool[] [FALSE, FALSE, FALSE, FALSE, FALSE, FALSE, FALSE, FALSE, FALSE, FALSE, FALSE, FALSE, FALSE, FALSE, FALSE, FALSE, FALSE, FALSE, FALSE, FALSE, FALSE, FALSE, FALSE, FALSE] ("24H周期设置") -> [w406]
          n324 = Replace Array Subset(array=w406, new element=TRUE ("新元素/子数组"), index=w405) -> (w403:bool[])
        }
        n325 = for {
          tunnel: w373 -> [w401] mode=indexing
          shift-right: [w399] -> w374
          shift-left: bool[] [FALSE, FALSE, FALSE, FALSE, FALSE, FALSE, FALSE, FALSE, FALSE, FALSE, FALSE, FALSE, FALSE, FALSE, FALSE, FALSE, FALSE, FALSE, FALSE, FALSE, FALSE, FALSE, FALSE, FALSE] ("24H周期设置") -> [w402]
          n326 = Replace Array Subset(array=w402, new element=TRUE ("新元素/子数组"), index=w401) -> (w399:bool[])
        }
        n327 = Get Date/Time In Seconds() -> (seconds since 1Jan1904=w386:timestamp)
        n328 = Get Date/Time In Seconds() -> (seconds since 1Jan1904=w366:timestamp)
        n329 = global write "系统设置全局变量.vi" "24H周期设置"(w395) -> ()
        n330 = Seconds To Date/Time(time stamp (now)=w386) -> (date time rec=w385:T9)  [unwired: 1 in]
        n331 = Seconds To Date/Time(time stamp (now)=w366) -> (date time rec=w367:T9)  [unwired: 1 in]
        n332 = Array To Cluster(array=w395) -> (cluster=w375:T14)
        n333 = local write "24H周期设置"(w375) -> ()
        n334 = Unbundle By Name(w385) -> ("时"=w382:i32, "分"=w384:i32)
        n335 = Unbundle By Name(w367) -> ("时"=w370:i32, "分"=w368:i32)
        n336 = Index Array(array=w378, index=w382) -> (element=w381:bool)
        n337 = Index Array(array=w374, index=w370) -> (element=w371:bool)
        n338 = Equal To 0?(x=w384) -> (x = 0?=w383:bool)
        n339 = Equal To 0?(x=w368) -> (x = 0?=w369:bool)
        n340 = And(x=w381, y=w383) -> (x .and. y?=w376:bool)
        n341 = And(x=w371, y=w369) -> (x .and. y?=w364:bool)
      }
      frame "流量设定" {
        n342 = global read "流量计全局变量.vi" "总流量"() -> (w419:dbl)
        n343 = feedback #1() -> (w416:i16)  [unwired: 1 in]
        n344 = Greater Or Equal?(x=w419, y="流量阈值") -> (x >= y?=w414:bool)
        n345 = Increment(x=w416) -> (x+1=w415:i16)
        n346 = Select(t=w415, s=w414, f=i16 0) -> (s? t:f=w413:i16)
        n347 = feedback-in #1(w413) -> ()
        n348 = Greater Or Equal?(x=w413, y="时间阈值") -> (x >= y?=w411:bool)
      }
    }
    n349 = call "周期设置.vi"("seconds since 1Jan1904"=w341, "质控启动日期"="质控启动日期", "跨度核查时间"="跨度核查时间", "零点核查时间"="空白核查时间", "运行模式"="运行模式") -> ("跨度核查启动命令"=w332:bool, "零点核查启动命令"=w333:bool, "水样测试启动命令"=w342:bool)  [unwired: 4 in]
    n350 = Or(x=w332, y=w333) -> (x .or. y?=w346:bool)
    n351 = Or(x=w333, y=w332) -> (x .or. y?=w334:bool)
    n352 = call <vilib>:"Boolean Crossing PtByPt.vi"("direction"=enum16{"either", "false-true", "true-false"}."false-true", "input"=w346) -> ("crossing"=w340:bool)  [unwired: 1 in]
    n353 = case shown="True" w340 {
      tunnel: w332 -> [_ w426]
      tunnel: w338 -> [_ w423]
      frame False {
      }
      frame True {
        n354 = local read "自动运行启动参数"() -> (w420:T2)
        n355 = Select(t=T16."跨度核查" ("元素"), s=w426, f=T16."零点核查" ("元素")) -> (s? t:f=w422:T16)
        n356 = Bundle("元素"=w422, "自动运行启动参数"=w420) -> (w421:T20)  [unwired: 1 in]
        n357 = Send Notification ("发送通知")(notification=w421, notifier=w423) -> ()  [unwired: 1 in, 2 out]
      }
    }
    n358 = Compound Arithmetic op=OR ("复合运算")(w336, w335, w329) -> (w348:bool)
    n359 = And(x=w348, y=w342) -> (x .and. y?=w349:bool)
    n360 = call <vilib>:"Boolean Crossing PtByPt.vi"("direction"=enum16{"either", "false-true", "true-false"}."false-true", "input"=w349) -> ("crossing"=w337:bool)  [unwired: 1 in]
    n361 = case shown="True" w337 {
      tunnel: w353 -> [_ w431]
      tunnel: w334 -> [_ w427]
      tunnel: w336 -> [_ w430]
      tunnel: w335 -> [_ w429]
      tunnel: w347 -> [_ w428]
      frame False {
      }
      frame True {
        n362 = flat-sequence {
          tunnel: w431 -> [w432]
          tunnel: w427 -> [w458]
          tunnel: w430 -> [w449]
          tunnel: w429 -> [w448]
          tunnel: w428 -> [w447]
          frame #0 {
            n363 = Cancel Notification(0:w432) -> ()  [unwired: 1 in, 3 out]
          }
          frame #1 {
            # "True"
            n364 = Format Date/Time String() -> (date/time string=→"最近一次启动时间":string)  [unwired: 3 in]
            n365 = Unbundle By Name("自动运行启动参数") -> ("多参数"=w452:bool, "CODmn"=w453:bool, "总磷"=w454:bool, "氨氮"=w455:bool, "CODCr"=w456:bool, "总氮"=w444:bool, "氟化物"=w440:bool, "超标留样"=w441:bool, "重金属"=w438:bool, "挥发酚"=w436:bool, "综合生物毒性"=w434:bool)
            n366 = And(x=w449, y=w452) -> (x .and. y?=w450:bool)
            n367 = case shown="False" w458 {
              tunnel: [w480 _] -> w462
              tunnel: [w478 _] -> w461
              tunnel: [w474 _] -> w460
              tunnel: [w475 _] -> w459
              tunnel: w456 -> [w473 _]
              tunnel: w455 -> [w476 _]
              tunnel: w454 -> [w477 _]
              tunnel: w453 -> [w479 _]
              tunnel: [w471 _] -> w451
              tunnel: w444 -> [w472 _]
              tunnel: w441 -> [w470 _]
              tunnel: [w470 _] -> w442
              tunnel: w448 -> [w481 _]
              tunnel: w440 -> [w469 _]
              tunnel: [w468 _] -> w439
              tunnel: w438 -> [w467 _]
              tunnel: [w467 _] -> w437
              tunnel: w436 -> [w466 _]
              tunnel: [w465 _] -> w435
              tunnel: w434 -> [w464 _]
              tunnel: [w463 _] -> w433
              frame False {
                n368 = case shown="False" w481 {
                  tunnel: [_ w489] -> w480
                  tunnel: w479 -> [_ w489]
                  tunnel: [_ w488] -> w478
                  tunnel: w477 -> [_ w488]
                  tunnel: [_ w487] -> w475
                  tunnel: w476 -> [_ w487]
                  tunnel: [_ w486] -> w474
                  tunnel: w473 -> [_ w486]
                  tunnel: [_ w485] -> w471
                  tunnel: w472 -> [_ w485]
                  tunnel: [_ w484] -> w468
                  tunnel: w469 -> [_ w484]
                  tunnel: w466 -> [_ w483]
                  tunnel: [_ w483] -> w465
                  tunnel: w464 -> [_ w482]
                  tunnel: [_ w482] -> w463
                  frame False {
                  }
                  frame True {
                  }
                }
              }
              frame True {
              }
            }
            n369 = Bundle By Name(cluster=T5 {"测试模式"=enum."水样测试", "参数启用"={"氨氮"=FALSE, "总磷"=FALSE, "总氮"=FALSE, "多参数"=FALSE, "CODmn"=FALSE, "CODCr"=FALSE, "氟化物"=FALSE, "超标留样"=FALSE, "重金属"=FALSE, "挥发酚"=FALSE, "综合生物毒性"=FALSE}} ("参数"), "参数启用.多参数"=w450, "参数启用.CODmn"=w462, "参数启用.总磷"=w461, "参数启用.氨氮"=w459, "参数启用.CODCr"=w460, "参数启用.总氮"=w451, "参数启用.氟化物"=w439, "参数启用.超标留样"=w442, "参数启用.重金属"=w437, "参数启用.挥发酚"=w435, "参数启用.综合生物毒性"=w433) -> (w446:T5)
            n370 = Enqueue Element(queue=w447, element=w446) -> ()  [unwired: 2 in, 3 out]
          }
        }
      }
    }
    "选项卡控件" <- "周期设置"
  }
